vi "Test_Tool.vi"(7 "String":string, 8 "error in":errorcluster, 9 "Simulate Error?":bool, 10 "max":dbl, 11 "min":dbl) -> (0 "error out":errorcluster, 2 "Echo String":string, 3 "random":dbl)   [LabVIEW 2025, in "MCP Server.lvlib"]
doc: "This is a test tool, it can return a random number within a given range. It can also output a simulated error and echo a string back that you input."
uses:
  MCP Server.lvlib
  <vilib>/Utility/error.llb/Error Cluster From Error Code.vi
  <vilib>/ErrorRing/Error Ring.xnode
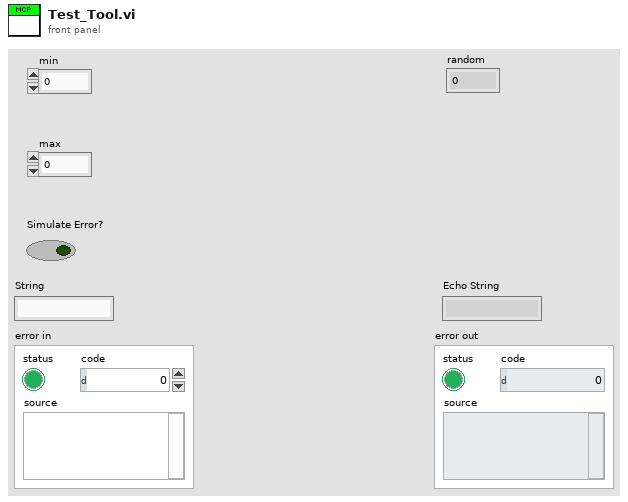
[diagram p1: front panel]
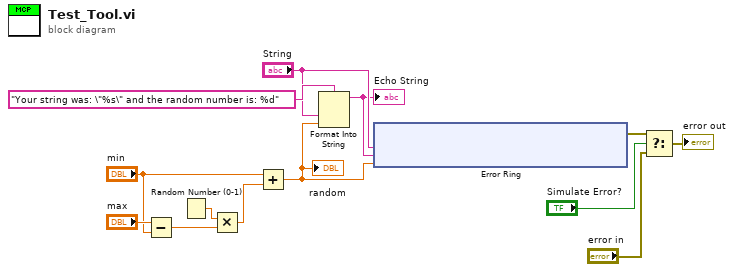
[diagram p0: block diagram]
diagram:
  n1 = Subtract(x="max", y="min") -> (x-y=w11:dbl)
  n2 = Random Number (0-1)() -> (number: 0 to 1=w12:dbl)
  n3 = Multiply(x=w12, y=w11) -> (x*y=w9:dbl)
  n4 = Add(x="min", y=w9) -> (x+y=w1:dbl)
  "random" <- w1
  n5 = Format Into String(format string="Your string was: \"%s\" and the random number is: %d", "String", w1) -> (resulting string=w2:string)  [unwired: 2 in, 1 out]
  "Echo String" <- w2
  n6 = xnode "Error Ring"("parameter 0"="String", "parameter 1"=w2, "parameter 2"=w1) -> ("error out"=w5:errorcluster)
  n7 = Select(t=w5, s="Simulate Error?", f="error in") -> (s? t:f=→"error out":errorcluster)
